vi "G#Object_Create.vi"(0 "reference in":refnum<class "MyG#SubClass.lvclass">, 3 "control values":variant[](array[variant]), 5 "error in (no error)":errorcluster) -> (14 "reference out":refnum<class "MyG#SubClass.lvclass">, 19 "error out":errorcluster)   [LabVIEW 2017, in "MyG#SubClass.lvclass"]
uses:
  MyG#SubClass.lvclass
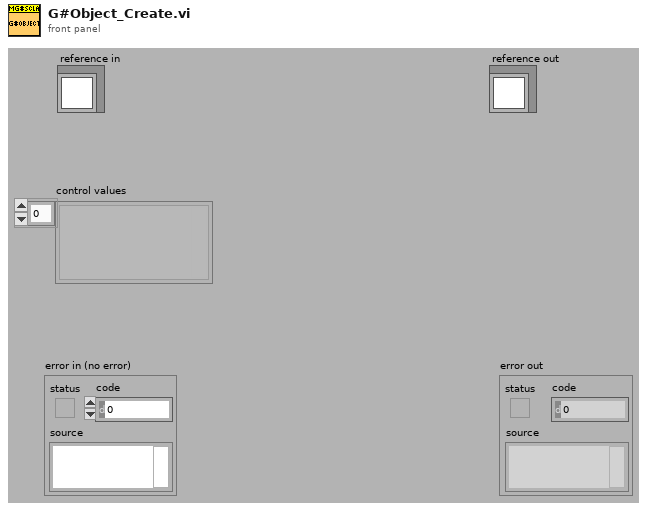
[diagram p1: front panel]
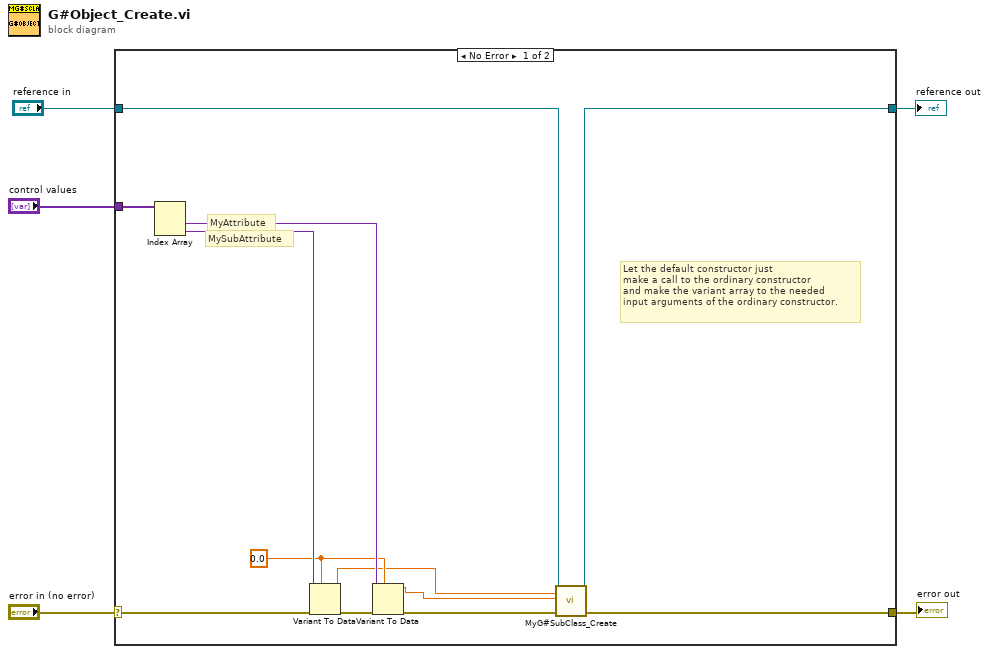
[diagram p0: block diagram]
diagram:
  n1 = case shown="No Error" "error in (no error)" {
    selector: "error in (no error)" -> [w13 w19]
    tunnel: [w17 w19] -> w4
    tunnel: [w15 w18] -> w2
    tunnel: "reference in" -> [w16 w18]
    tunnel: "control values" -> [w14 _]
    frame No Error {
      w8 = 0.0 ("MyAttribute")
      # "MySubAttribute"
      # "MyAttribute"
      # "Let the default constructor just\nmake a call to the ordinary constructor\nand make the variant array to the needed\ninput arguments of the ordinary constructor."
      n2 = Index Array(array=w14) -> (element #1=w9:variant, element #2=w10:variant)  [unwired: 2 in]
      n3 = Variant To Data(error in=w13, type=w8, Variant=w10) -> (data=w7:dbl, error out=w12:errorcluster)
      n4 = Variant To Data(error in=w12, type=w8, Variant=w9) -> (data=w6:dbl, error out=w11:errorcluster)
      n5 = call "MyG#SubClass_Create.vi"("reference in"=w16, "MySubAttribute"=w7, "MyAttribute"=w6, "error in (no error)"=w11) -> ("reference out"=w15:refnum<class "MyG#SubClass.lvclass">, "error out"=w17:errorcluster)  [unwired: 14 in]
    }
    frame Error {
    }
  }
  "error out" <- w4
  "reference out" <- w2
